vi "MeasLeakRate04.vi"() -> ()   [LabVIEW 2011]
panel:
  in  "reset":bool
  in  "# points to watch":i32=60
  out "leak rate (Torr/min)":string
  out "S20":dbl
  out "S11":dbl
  out "S10":dbl
  out "S01":dbl
  out "S00":dbl
  out "A11":dbl[](array[numeric])
  out "P":dbl
  in  "first":bool=TRUE
  out "A20":dbl[](array[numeric])
  out "A10":dbl[](array[numeric])
  out "A01":dbl[](array[numeric])
  out "A00":dbl[](array[numeric])
  in  "interval (s)":dbl=0.5
  in  "stop":bool
  out "P(Torr)":string
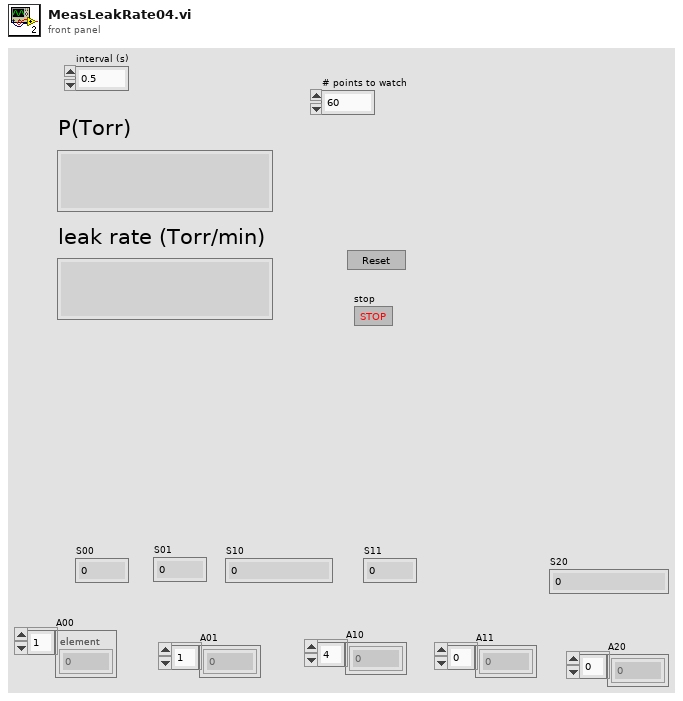
[diagram p1: front panel]
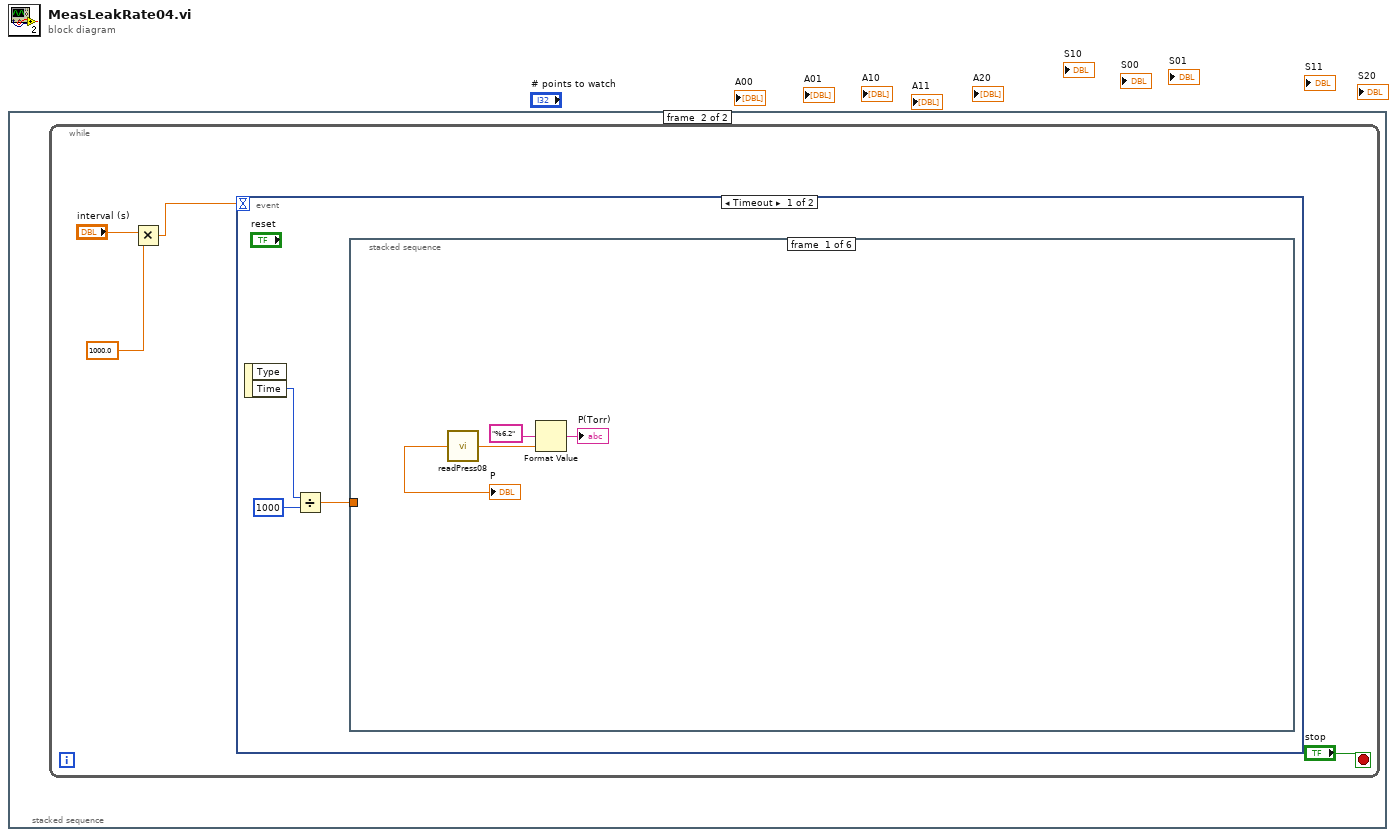
[diagram p0: block diagram]
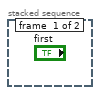
[diagram p2: hidden frame]
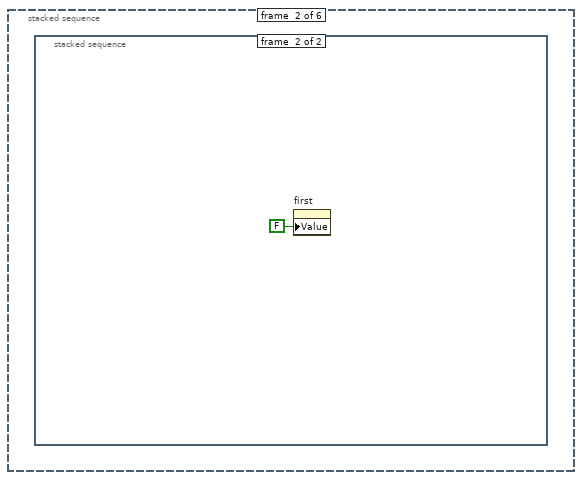
[diagram p3: hidden frame]
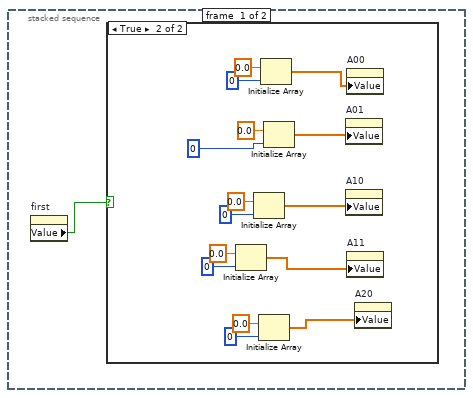
[diagram p4: hidden frame]
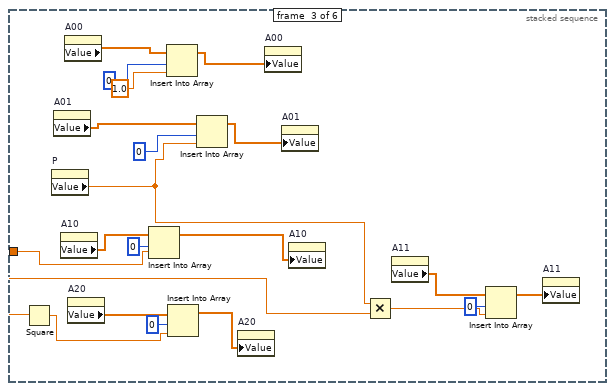
[diagram p6: hidden frame]
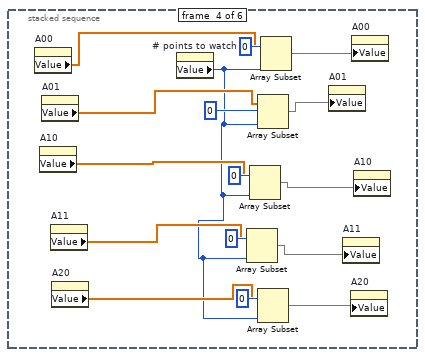
[diagram p7: hidden frame]
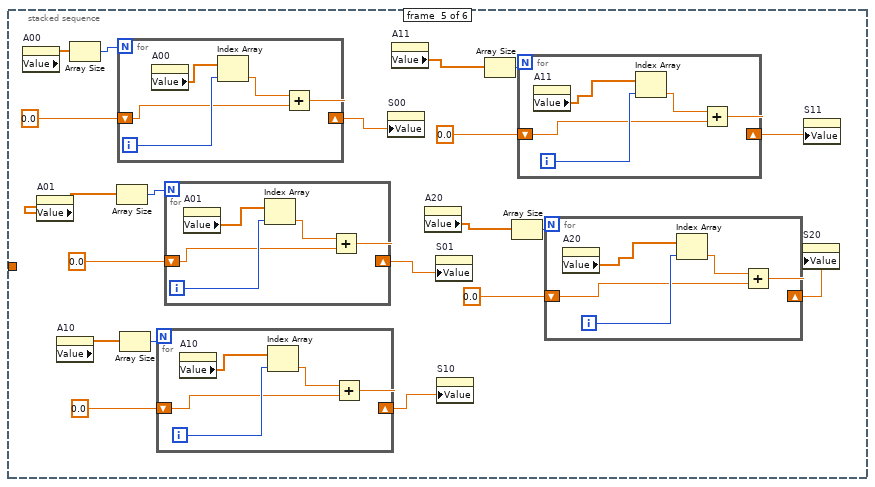
[diagram p8: hidden frame]
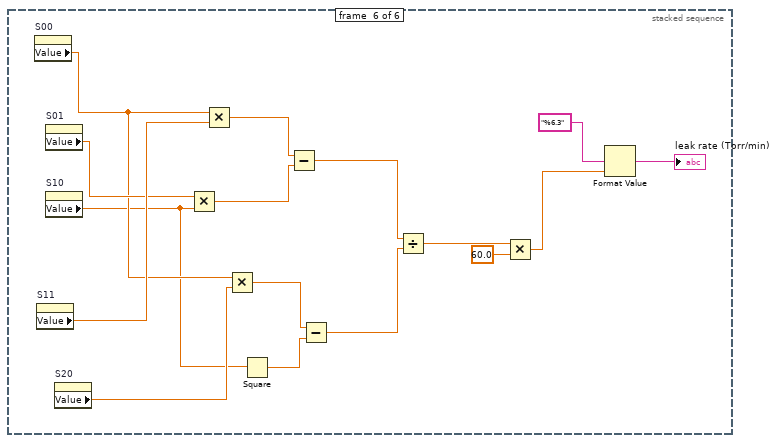
[diagram p9: hidden frame]
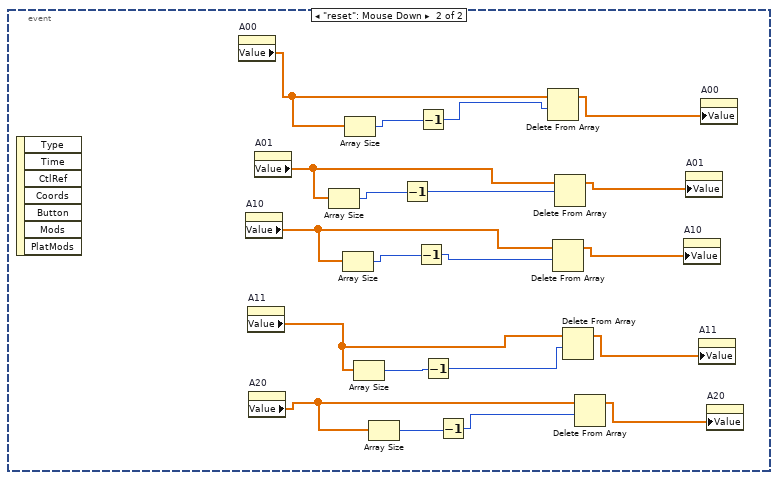
[diagram p10: hidden frame]
diagram:
  n1 = stacked-sequence {
    frame #0 {
    }
    frame #1 {
      n2 = while {
        stop <- "stop" stop-if-true
        n3 = Multiply(x="interval (s)", y=1000.0) -> (x*y=w2:dbl)
        n4 = event shown="[0] Timeout" {
          selector: _ -> [_ _]
          dyn-events: _ -> [_ _]
          timeout: w2 -> [_ _]
          event Timeout {
            n5 = event-data() -> ("Time"=w7:u32)  [unwired: 1 in, 1 out]
            n6 = Divide(x=w7, y=u32 1000) -> (x/y=w5:dbl)
            n7 = stacked-sequence {
              tunnel: w5 -> [_ _ w37 _ _ _]
              frame #0 {
                n8 = call "readPress08.vi"() -> ("P"=w9:dbl)
                "P" <- w9
                n9 = Format Value(format string="%6.2", value (0)=w9) -> (output string=→"P(Torr)":string)  [unwired: 1 in]
              }
              frame #1 {
                n10 = stacked-sequence {
                  frame #0 {
                    n11 = property on="first" class="Bool (strict)"() -> ("Value"=w11:bool)  [unwired: 2 in, 2 out]
                    n12 = case shown="True" w11 {
                      frame False {
                      }
                      frame True {
                        n13 = Initialize Array(0.0 ("element"), 0 ("dimension size")) -> (w14:dbl[])
                        n14 = Initialize Array(0.0 ("element"), 0 ("dimension size")) -> (w15:dbl[])
                        n15 = Initialize Array(0.0 ("element"), 0 ("dimension size")) -> (w13:dbl[])
                        n16 = Initialize Array(0.0 ("element"), 0 ("dimension size")) -> (w12:dbl[])
                        n17 = Initialize Array(0.0 ("element"), 0 ("dimension size")) -> (w16:dbl[])
                        n18 = property on="A01" class="Arr (strict)"("Value"=w16) -> ()  [unwired: 2 in, 2 out]
                        n19 = property on="A10" class="Arr (strict)"("Value"=w15) -> ()  [unwired: 2 in, 2 out]
                        n20 = property on="A00" class="Arr (strict)"("Value"=w12) -> ()  [unwired: 2 in, 2 out]
                        n21 = property on="A11" class="Arr (strict)"("Value"=w14) -> ()  [unwired: 2 in, 2 out]
                        n22 = property on="A20" class="Arr (strict)"("Value"=w13) -> ()  [unwired: 2 in, 2 out]
                      }
                    }
                  }
                  frame #1 {
                    n23 = property on="first" class="Bool (strict)"("Value"=FALSE ("first")) -> ()  [unwired: 2 in, 2 out]
                  }
                }
              }
              frame #2 {
                n24 = Square(x=w37) -> (x^2=w38:dbl)
                n25 = property on="P" class="DigNum (strict)"() -> ("Value"=w36:dbl)  [unwired: 2 in, 2 out]
                n26 = property on="A01" class="Arr (strict)"() -> ("Value"=w43:dbl[])  [unwired: 2 in, 2 out]
                n27 = property on="A10" class="Arr (strict)"() -> ("Value"=w42:dbl[])  [unwired: 2 in, 2 out]
                n28 = property on="A00" class="Arr (strict)"() -> ("Value"=w45:dbl[])  [unwired: 2 in, 2 out]
                n29 = property on="A20" class="Arr (strict)"() -> ("Value"=w40:dbl[])  [unwired: 2 in, 2 out]
                n30 = Insert Into Array(array=w42, index=0, new element=w37) -> (w30:dbl[])
                n31 = Insert Into Array(array=w45, index=0, new element=1.0 ("new element/subarray")) -> (w32:dbl[])
                n32 = Insert Into Array(array=w40, index=0, new element=w38) -> (w31:dbl[])
                n33 = Insert Into Array(array=w43, index=0, new element=w36) -> (w28:dbl[])
                n34 = property on="A20" class="Arr (strict)"("Value"=w31) -> ()  [unwired: 2 in, 2 out]
                n35 = property on="A00" class="Arr (strict)"("Value"=w32) -> ()  [unwired: 2 in, 2 out]
                n36 = property on="A01" class="Arr (strict)"("Value"=w28) -> ()  [unwired: 2 in, 2 out]
                n37 = property on="A10" class="Arr (strict)"("Value"=w30) -> ()  [unwired: 2 in, 2 out]
                n38 = Multiply(x=w36, y=w37) -> (x*y=w34:dbl)
                n39 = property on="A11" class="Arr (strict)"() -> ("Value"=w35:dbl[])  [unwired: 2 in, 2 out]
                n40 = Insert Into Array(array=w35, index=0, new element=w34) -> (w29:dbl[])
                n41 = property on="A11" class="Arr (strict)"("Value"=w29) -> ()  [unwired: 2 in, 2 out]
              }
              frame #3 {
                n42 = property on="A00" class="Arr (strict)"() -> ("Value"=w60:dbl[])  [unwired: 2 in, 2 out]
                n43 = property on="A10" class="Arr (strict)"() -> ("Value"=w54:dbl[])  [unwired: 2 in, 2 out]
                n44 = property on="A01" class="Arr (strict)"() -> ("Value"=w55:dbl[])  [unwired: 2 in, 2 out]
                n45 = property on="A11" class="Arr (strict)"() -> ("Value"=w53:dbl[])  [unwired: 2 in, 2 out]
                n46 = property on="A20" class="Arr (strict)"() -> ("Value"=w62:dbl[])  [unwired: 2 in, 2 out]
                n47 = property on="# points to watch" class="DigNum (strict)"() -> ("Value"=w48:i32)  [unwired: 2 in, 2 out]
                n48 = Array Subset(array=w53, index=0, length=w48) -> (w50:dbl[])
                n49 = Array Subset(array=w54, index=0, length=w48) -> (w51:dbl[])
                n50 = Array Subset(array=w55, index=0, length=w48) -> (w52:dbl[])
                n51 = Array Subset(array=w62, index=0, length=w48) -> (w49:dbl[])
                n52 = Array Subset(array=w60, index=0, length=w48) -> (w59:dbl[])
                n53 = property on="A01" class="Arr (strict)"("Value"=w52) -> ()  [unwired: 2 in, 2 out]
                n54 = property on="A11" class="Arr (strict)"("Value"=w50) -> ()  [unwired: 2 in, 2 out]
                n55 = property on="A20" class="Arr (strict)"("Value"=w49) -> ()  [unwired: 2 in, 2 out]
                n56 = property on="A00" class="Arr (strict)"("Value"=w59) -> ()  [unwired: 2 in, 2 out]
                n57 = property on="A10" class="Arr (strict)"("Value"=w51) -> ()  [unwired: 2 in, 2 out]
              }
              frame #4 {
                n58 = property on="A00" class="Arr (strict)"() -> ("Value"=w82:dbl[])  [unwired: 2 in, 2 out]
                n59 = property on="A01" class="Arr (strict)"() -> ("Value"=w78:dbl[])  [unwired: 2 in, 2 out]
                n60 = property on="A10" class="Arr (strict)"() -> ("Value"=w75:dbl[])  [unwired: 2 in, 2 out]
                n61 = Array Size(array=w82) -> (size(s)=w83:i32)
                n62 = Array Size(array=w78) -> (size(s)=w80:i32)
                n63 = for {
                  N: w83 -> [_]
                  shift-right: [w104] -> w68
                  shift-left: 0.0 -> [w105]
                  i -> [w107]
                  n64 = property on="A00" class="Arr (strict)"() -> ("Value"=w108:dbl[])  [unwired: 2 in, 2 out]
                  n65 = Index Array(array=w108, index=w107) -> (element=w106:dbl)
                  n66 = Add(x=w106, y=w105) -> (x+y=w104:dbl)
                }
                n67 = Array Size(array=w75) -> (size(s)=w77:i32)
                n68 = for {
                  N: w77 -> [_]
                  shift-right: [w95] -> w67
                  shift-left: 0.0 -> [w96]
                  i -> [w98]
                  n69 = property on="A10" class="Arr (strict)"() -> ("Value"=w94:dbl[])  [unwired: 2 in, 2 out]
                  n70 = Index Array(array=w94, index=w98) -> (element=w97:dbl)
                  n71 = Add(x=w97, y=w96) -> (x+y=w95:dbl)
                }
                n72 = for {
                  N: w80 -> [_]
                  shift-right: [w100] -> w66
                  shift-left: 0.0 -> [w101]
                  i -> [w103]
                  n73 = property on="A01" class="Arr (strict)"() -> ("Value"=w99:dbl[])  [unwired: 2 in, 2 out]
                  n74 = Index Array(array=w99, index=w103) -> (element=w102:dbl)
                  n75 = Add(x=w102, y=w101) -> (x+y=w100:dbl)
                }
                n76 = property on="S00" class="DigNum (strict)"("Value"=w68) -> ()  [unwired: 2 in, 2 out]
                n77 = property on="A11" class="Arr (strict)"() -> ("Value"=w72:dbl[])  [unwired: 2 in, 2 out]
                n78 = property on="A20" class="Arr (strict)"() -> ("Value"=w69:dbl[])  [unwired: 2 in, 2 out]
                n79 = property on="S01" class="DigNum (strict)"("Value"=w66) -> ()  [unwired: 2 in, 2 out]
                n80 = property on="S10" class="DigNum (strict)"("Value"=w67) -> ()  [unwired: 2 in, 2 out]
                n81 = Array Size(array=w72) -> (size(s)=w74:i32)
                n82 = Array Size(array=w69) -> (size(s)=w71:i32)
                n83 = for {
                  N: w74 -> [_]
                  shift-right: [w90] -> w65
                  shift-left: 0.0 -> [w91]
                  i -> [w93]
                  n84 = property on="A11" class="Arr (strict)"() -> ("Value"=w89:dbl[])  [unwired: 2 in, 2 out]
                  n85 = Index Array(array=w89, index=w93) -> (element=w92:dbl)
                  n86 = Add(x=w92, y=w91) -> (x+y=w90:dbl)
                }
                n87 = for {
                  N: w71 -> [_]
                  shift-right: [w85] -> w64
                  shift-left: 0.0 -> [w86]
                  i -> [w88]
                  n88 = property on="A20" class="Arr (strict)"() -> ("Value"=w84:dbl[])  [unwired: 2 in, 2 out]
                  n89 = Index Array(array=w84, index=w88) -> (element=w87:dbl)
                  n90 = Add(x=w87, y=w86) -> (x+y=w85:dbl)
                }
                n91 = property on="S20" class="DigNum (strict)"("Value"=w64) -> ()  [unwired: 2 in, 2 out]
                n92 = property on="S11" class="DigNum (strict)"("Value"=w65) -> ()  [unwired: 2 in, 2 out]
              }
              frame #5 {
                n93 = property on="S00" class="DigNum (strict)"() -> ("Value"=w120:dbl)  [unwired: 2 in, 2 out]
                n94 = property on="S11" class="DigNum (strict)"() -> ("Value"=w124:dbl)  [unwired: 2 in, 2 out]
                n95 = property on="S01" class="DigNum (strict)"() -> ("Value"=w123:dbl)  [unwired: 2 in, 2 out]
                n96 = property on="S10" class="DigNum (strict)"() -> ("Value"=w118:dbl)  [unwired: 2 in, 2 out]
                n97 = property on="S20" class="DigNum (strict)"() -> ("Value"=w119:dbl)  [unwired: 2 in, 2 out]
                n98 = Multiply(x=w123, y=w118) -> (x*y=w121:dbl)
                n99 = Multiply(x=w120, y=w124) -> (x*y=w122:dbl)
                n100 = Multiply(x=w120, y=w119) -> (x*y=w117:dbl)
                n101 = Square(x=w118) -> (x^2=w116:dbl)
                n102 = Subtract(x=w122, y=w121) -> (x-y=w115:dbl)
                n103 = Subtract(x=w117, y=w116) -> (x-y=w114:dbl)
                n104 = Divide(x=w115, y=w114) -> (x/y=w113:dbl)
                n105 = Multiply(x=w113, y=60.0) -> (x*y=w109:dbl)
                n106 = Format Value(format string="%6.3", value (0)=w109) -> (output string=→"leak rate (Torr/min)":string)  [unwired: 1 in]
              }
            }
          }
          event "reset": Mouse Down {
            n107 = event-data() -> ()  [unwired: 1 in, 7 out]
            n108 = property on="A00" class="Arr (strict)"() -> ("Value"=w144:dbl[])  [unwired: 2 in, 2 out]
            n109 = property on="A10" class="Arr (strict)"() -> ("Value"=w137:dbl[])  [unwired: 2 in, 2 out]
            n110 = property on="A11" class="Arr (strict)"() -> ("Value"=w134:dbl[])  [unwired: 2 in, 2 out]
            n111 = property on="A20" class="Arr (strict)"() -> ("Value"=w131:dbl[])  [unwired: 2 in, 2 out]
            n112 = property on="A01" class="Arr (strict)"() -> ("Value"=w140:dbl[])  [unwired: 2 in, 2 out]
            n113 = Array Size(array=w140) -> (size(s)=w139:i32)
            n114 = Array Size(array=w137) -> (size(s)=w136:i32)
            n115 = Array Size(array=w144) -> (size(s)=w142:i32)
            n116 = Array Size(array=w134) -> (size(s)=w133:i32)
            n117 = Array Size(array=w131) -> (size(s)=w130:i32)
            n118 = Decrement(x=w139) -> (x-1=w138:i32)
            n119 = Decrement(x=w136) -> (x-1=w135:i32)
            n120 = Decrement(x=w142) -> (x-1=w141:i32)
            n121 = Decrement(x=w133) -> (x-1=w132:i32)
            n122 = Decrement(x=w130) -> (x-1=w129:i32)
            n123 = Delete From Array(array=w144, length=w141) -> (array with subset deleted=w143:dbl[])  [unwired: 1 in, 1 out]
            n124 = Delete From Array(array=w137, length=w135) -> (array with subset deleted=w127:dbl[])  [unwired: 1 in, 1 out]
            n125 = Delete From Array(array=w140, length=w138) -> (array with subset deleted=w128:dbl[])  [unwired: 1 in, 1 out]
            n126 = Delete From Array(array=w134, length=w132) -> (array with subset deleted=w126:dbl[])  [unwired: 1 in, 1 out]
            n127 = Delete From Array(array=w131, length=w129) -> (array with subset deleted=w125:dbl[])  [unwired: 1 in, 1 out]
            n128 = property on="A10" class="Arr (strict)"("Value"=w127) -> ()  [unwired: 2 in, 2 out]
            n129 = property on="A01" class="Arr (strict)"("Value"=w128) -> ()  [unwired: 2 in, 2 out]
            n130 = property on="A11" class="Arr (strict)"("Value"=w126) -> ()  [unwired: 2 in, 2 out]
            n131 = property on="A00" class="Arr (strict)"("Value"=w143) -> ()  [unwired: 2 in, 2 out]
            n132 = property on="A20" class="Arr (strict)"("Value"=w125) -> ()  [unwired: 2 in, 2 out]
          }
        }
      }
    }
  }
